vi "soundcard.vi"() -> ()   [LabVIEW 2013]
uses:
  <vilib>/sound2/lvsound2.llb/Sampling Mode.ctl
  <vilib>/sound2/lvsound2.llb/Sound Data Format.ctl
  <vilib>/sound2/lvsound2.llb/Sound Output Write (DBL Single).vi
  <vilib>/Analysis/NI_AALBase.lvlib
panel:
  out "Numeric":i32=4
  in  "sound format":T1={"sample rate (S/s)"=44100.0, "number of channels"=2, "bits per sample"=16}
  in  "device ID":u32
  in  "number of samples/ch":i32=8820
  in  "sample mode":T2=1 items=["Finite Samples", "Continuous Samples"]
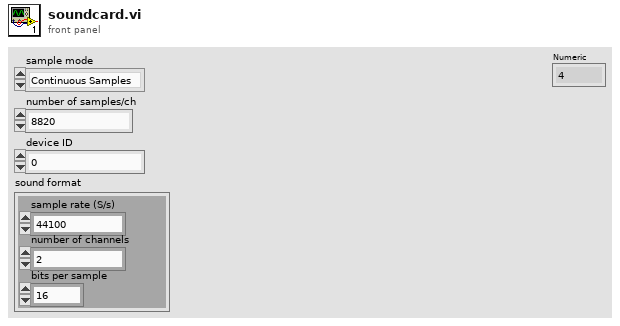
[diagram p1: front panel]
types:
  T1 = typedef "Sound Data Format.ctl" = cluster{"sample rate (S/s)":dbl, "number of channels":i32, "bits per sample":i32}
  T2 = typedef "Sampling Mode.ctl" = i32
  T3 = typedef "Sound Output Task ID.ctl" = u32
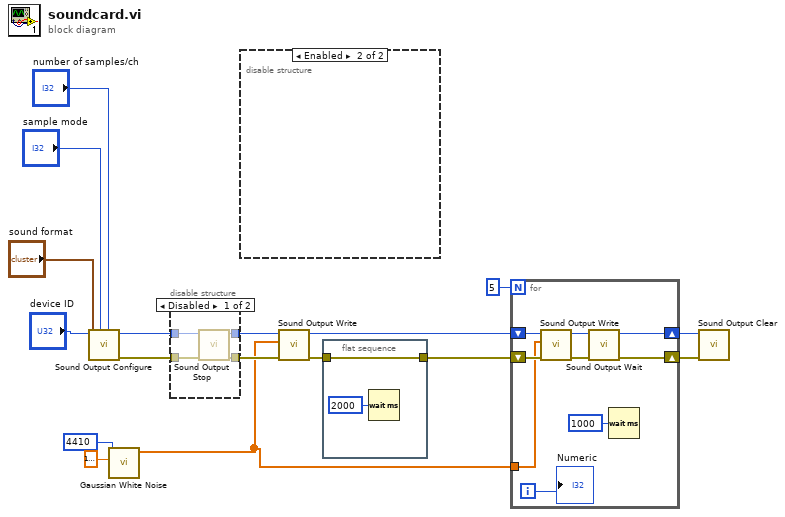
[diagram p0: block diagram]
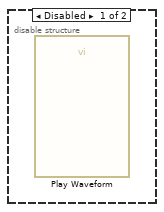
[diagram p3: hidden frame]
diagram:
  n1 = call <vilib>:"Sound Output Configure.vi"("number of samples/ch"="number of samples/ch", "sample mode"="sample mode", "sound format"="sound format", "device ID"="device ID") -> ("error out"=w6:errorcluster, "task ID"=w7:T3)  [unwired: 6 in]
  n2 = call <vilib>:"Gaussian White Noise.vi"("standard deviation"=1.0000000000000002, "samples"=4410) -> ("Gaussian noise pattern"=w1:dbl[])  [unwired: 8 in, 1 out]
  n3 = disable-structure shown="Disabled" {
    disable-tunnel: w7 -> [w21 w23]
    disable-tunnel: w6 -> [w20 w22]
    disable-tunnel: [w19 w23] -> w5
    disable-tunnel: [w18 w22] -> w4
    frame Disabled {
      n4 = call <vilib>:"Sound Output Stop.vi"("error in (no error)"=w20, "task ID"=w21) -> ("error out"=w18:errorcluster, "task ID out"=w19:T3)  [unwired: 8 in]
    }
    frame Enabled {
    }
  }
  n5 = disable-structure shown="Enabled" {
    frame Disabled {
      n6 = call "Play Waveform"() -> ()  [unwired: 19 in, 1 out]
    }
    frame Enabled {
    }
  }
  n7 = call-poly <vilib>:"Sound Output Write.vi"("error in (no error)"=w4, "data"=w1, "task ID"=w5) -> ("error out"=w11:errorcluster, "task ID out"=w3:T3)  [unwired: 7 in]
  n8 = flat-sequence {
    tunnel: w11 -> [w24]
    tunnel: [w24] -> w2
    frame #0 {
      n9 = Wait (ms)(milliseconds to wait=u32 2000) -> ()  [unwired: 1 out]
    }
  }
  n10 = for {
    N: 5 -> [_]
    shift-right: [w34] -> w9
    shift-left: w3 -> [w31]
    shift-right: [w33] -> w8
    shift-left: w2 -> [w28]
    tunnel: w1 -> [w27]
    i -> [w26]
    n11 = call-poly <vilib>:"Sound Output Write.vi"("error in (no error)"=w28, "data"=w27, "task ID"=w31) -> ("error out"=w29:errorcluster, "task ID out"=w30:T3)  [unwired: 7 in]
    n12 = call <vilib>:"Sound Output Wait.vi"("error in (no error)"=w29, "task ID"=w30) -> ("error out"=w33:errorcluster, "task ID out"=w34:T3)  [unwired: 8 in]
    n13 = Wait (ms)(milliseconds to wait=u32 1000) -> ()  [unwired: 1 out]
    "Numeric" <- w26
  }
  n14 = call <vilib>:"Sound Output Clear.vi"("error in (no error)"=w8, "task ID"=w9) -> ()  [unwired: 9 in, 1 out]
